vi "Configure Display.vi"(5 "Enable Display (Enable)":bool=TRUE, 7 "Display Mode (0:Measurement)":i32(ring) items=["Measurement", "Statistics", "Limit", "Scale Offset"], 8 "error in (no error)":errorcluster, 9 "Limit Display Mode (0:Number)":i32(ring) items=["Number", "Graph"], 10 "Statistics Display Mode (0:Mean)":i32(ring) items=["Mean", "Standard Deviation", "Minimum", "Maximum", "Delta"], 11 "VISA resource name":refnum<visa-resource-name>) -> (0 "error out":errorcluster, 3 "VISA resource name out":refnum<visa-resource-name>)   [LabVIEW 2020, in "Counter.lvlib" / "PICOTEST U62XXA series.lvlib"]
doc: "Configures all the settings that have to do with the display. It enables or disables the entire display, selects the Display mode, the Statistics display mode and the Limit Display mode."
uses:
  PICOTEST U62XXA series.lvlib
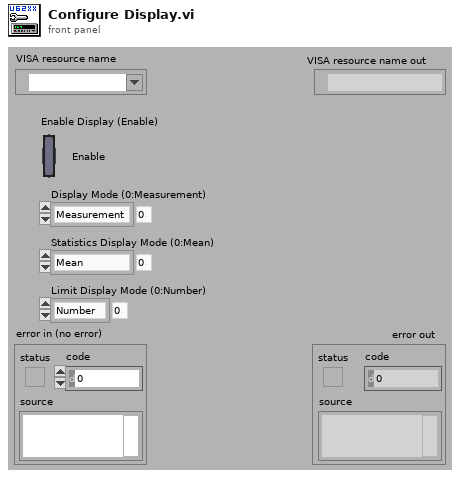
[diagram p1: front panel]
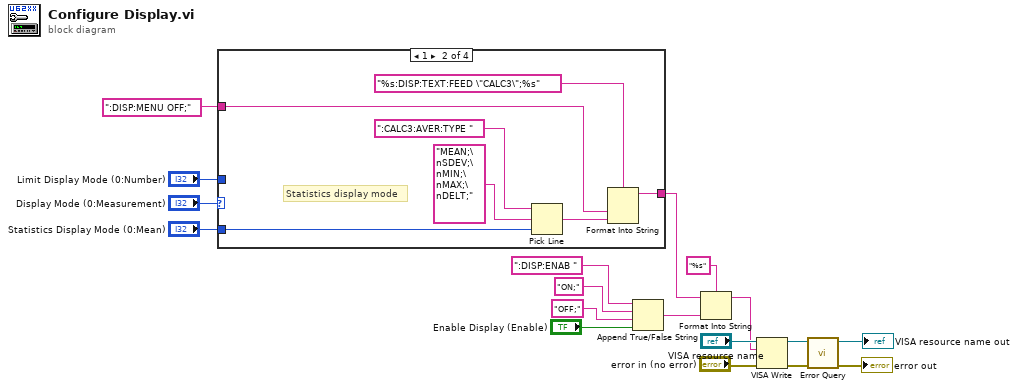
[diagram p0: block diagram]
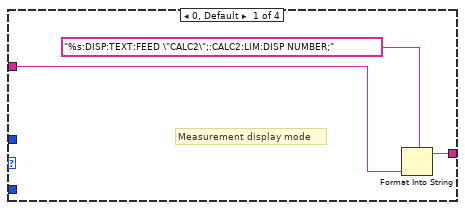
[diagram p2: hidden frame]
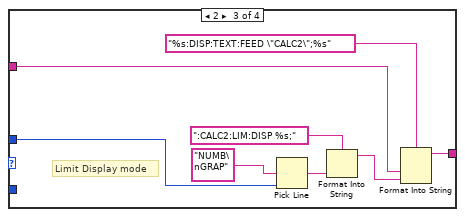
[diagram p3: hidden frame]
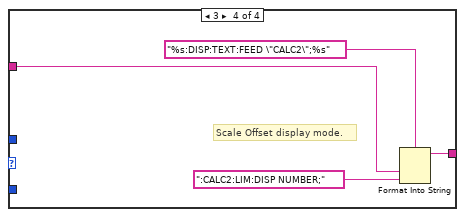
[diagram p4: hidden frame]
diagram:
  n1 = case shown="1" "Display Mode (0:Measurement)" {
    tunnel: ":DISP:MENU OFF;" -> [w20 w24 w30 w38]
    tunnel: [w21 w23 w32 w40] -> w2
    tunnel: "Statistics Display Mode (0:Mean)" -> [_ w26 _ _]
    tunnel: "Limit Display Mode (0:Number)" -> [_ _ w33 _]
    frame 0, Default {
      # "Measurement display mode"
      n2 = Format Into String(format string="%s:DISP:TEXT:FEED \"CALC2\";:CALC2:LIM:DISP NUMBER;", w20) -> (resulting string=w21:string)  [unwired: 2 in, 1 out]
    }
    frame 1 {
      # "Statistics display mode"
      n3 = Pick Line(string ("")=":CALC3:AVER:TYPE ", multi-line string="MEAN;\nSDEV;\nMIN;\nMAX;\nDELT;", line index=w26) -> (output string=w22:string)
      n4 = Format Into String(format string="%s:DISP:TEXT:FEED \"CALC3\";%s", w24, w22) -> (resulting string=w23:string)  [unwired: 2 in, 1 out]
    }
    frame 2 {
      # "Limit Display mode"
      n5 = Pick Line(multi-line string="NUMB\nGRAP" ("t"), line index=w33) -> (output string=w36:string)  [unwired: 1 in]
      n6 = Format Into String(format string=":CALC2:LIM:DISP %s;", w36) -> (resulting string=w29:string)  [unwired: 2 in, 1 out]
      n7 = Format Into String(format string="%s:DISP:TEXT:FEED \"CALC2\";%s", w30, w29) -> (resulting string=w32:string)  [unwired: 2 in, 1 out]
    }
    frame 3 {
      # "Scale Offset display mode."
      n8 = Format Into String(format string="%s:DISP:TEXT:FEED \"CALC2\";%s", w38, ":CALC2:LIM:DISP NUMBER;") -> (resulting string=w40:string)  [unwired: 2 in, 1 out]
    }
  }
  n9 = Append True/False String(1:"Enable Display (Enable)", 2:"OFF;" ("false string"), 3:"ON;" ("true string"), 4:":DISP:ENAB ") -> (0:w1:string)
  n10 = Format Into String(format string="%s", initial string=w2, w1) -> (resulting string=w3:string)  [unwired: 1 in, 1 out]
  n11 = VISA Write(VISA resource name="VISA resource name", write buffer=w3, error in (no error)="error in (no error)") -> (VISA resource name out=w10:refnum<visa-resource-name>, error out=w8:errorcluster)  [unwired: 1 out]
  n12 = call "Error Query.vi"("error in (no error)"=w8, "VISA resource name"=w10) -> ("error out"=→"error out":errorcluster, "VISA resource name out"=→"VISA resource name out":refnum<visa-resource-name>)  [unwired: 6 in, 2 out]
